vi "6.1.vi"   [LabVIEW 2017]
types:
  T1 = enum16{"open", "replace", "create", "open or create", "replace or create", "replace or create with confirmation"}
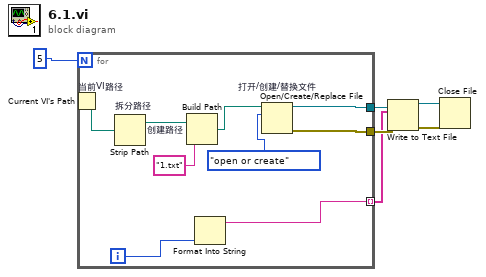
[diagram p0: block diagram]
diagram:
  n1 = for {
    N: 5 -> [_]
    tunnel: [w11] -> w3
    tunnel: [w10] -> w2
    tunnel: [w7] -> w1 mode=indexing
    i -> [w8]
    n2 = Current VI's Path "当前VI路径"() -> (path=w15:path)
    n3 = Strip Path "拆分路径"(path=w15) -> (stripped path=w14:path)  [unwired: 1 out]
    n4 = Build Path "创建路径"(base path=w14, name or relative path="1.txt") -> (appended path=w12:path)
    n5 = Format Into String(w8) -> (resulting string=w7:string)  [unwired: 3 in, 1 out]
    n6 = Open/Create/Replace File "打开/创建/替换文件"(file path (use dialog)=w12, operation (0:open)=T1."open or create" ("操作(0:open)")) -> (refnum out=w10:refnum<file>, error out=w11:errorcluster)  [unwired: 4 in, 1 out]
  }
  n7 = Write to Text File(file (use dialog)=w2, text=w1, error in=w3) -> (refnum out=w5:refnum<file>, error out=w4:errorcluster)  [unwired: 1 in, 1 out]
  n8 = Close File(refnum=w5, error in=w4) -> ()  [unwired: 2 out]
